vi "Configure Power.vi"(0 "VISA resource name":refnum<visa-resource-name>, 1 "Channel (1)":i32=1, 2 "Port (1)":i32=1, 3 "Port Coupling (T: On)":bool=TRUE, 5 "Power Level (0.0)":dbl format="%^.2g", 7 "Auto Power Range (F: Off)":bool, 9 "Power Range (0.0)":dbl format="%^.2g", 11 "error in (no error)":errorcluster, 12 "Power Slope (F: Off)":bool, 13 "Power Slope Coefficient (0.0)":dbl format="%^.2g") -> (4 "VISA resource name out":refnum<visa-resource-name>, 15 "error out":errorcluster)   [LabVIEW 2018, in "Agilent ENA Series.lvlib"]
doc: "Configures power settings.\n\n<b>Note:</b>\nThis VI is not supported by the E5063A model."
uses:
  Agilent ENA Series.lvlib
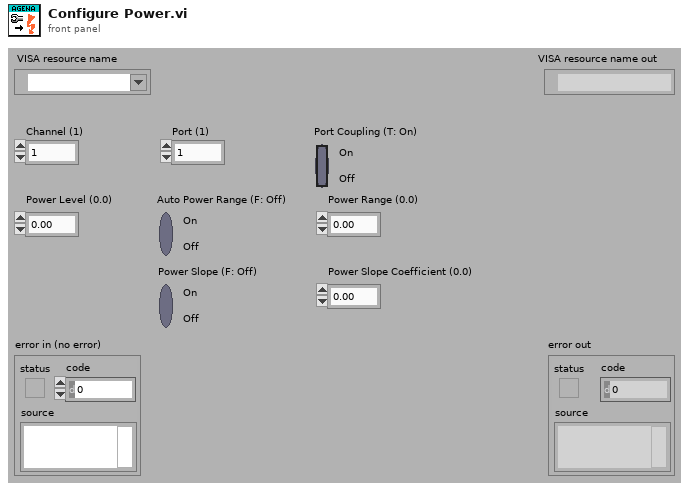
[diagram p1: front panel]
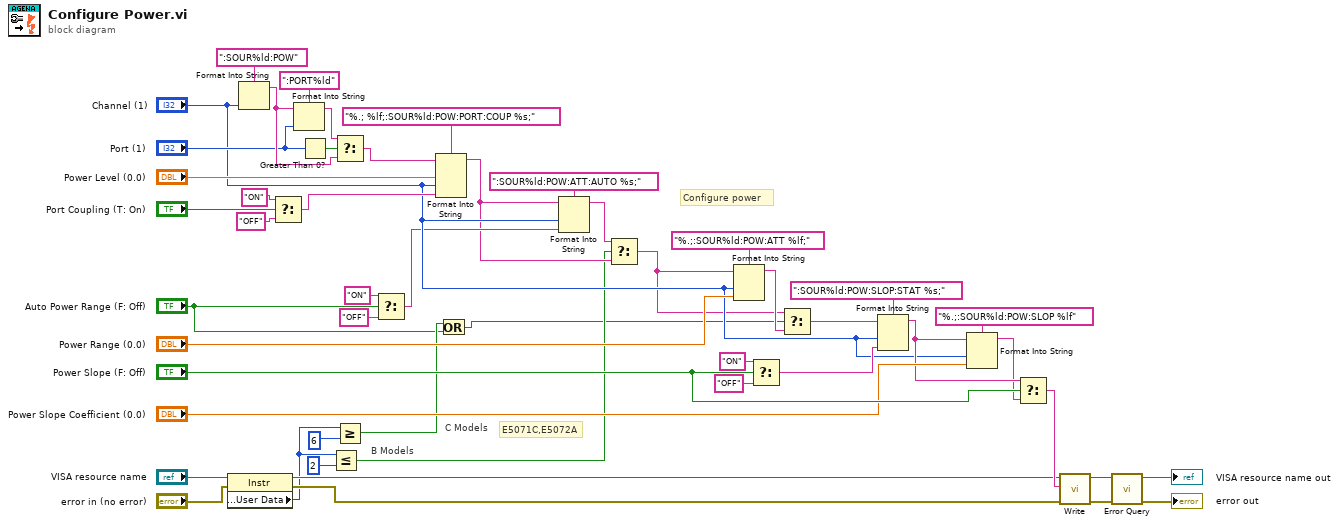
[diagram p0: block diagram]
diagram:
  # "E5071C,E5072A"
  # "Configure power"
  # "C Models"
  # "B Models"
  n1 = property class="Instr"(reference="VISA resource name", error in="error in (no error)") -> (reference out=w15:refnum<visa-resource-name>, error out=w14:errorcluster, "General Settings:User Data"=w2:u32)
  n2 = Format Into String(format string=":SOUR%ld:POW", "Channel (1)") -> (resulting string=w46:string)  [unwired: 2 in, 1 out]
  n3 = Select(t="ON", s="Port Coupling (T: On)", f="OFF") -> (s? t:f=w38:string)
  n4 = Format Into String(format string=":PORT%ld", initial string=w46, "Port (1)") -> (resulting string=w45:string)  [unwired: 1 in, 1 out]
  n5 = Greater Than 0?(x="Port (1)") -> (x > 0?=w47:bool)
  n6 = Less Or Equal?(x=w2, y=u32 2) -> (x <= y?=w7:bool)
  n7 = Select(t=w45, s=w47, f=w46) -> (s? t:f=w43:string)
  n8 = Greater Or Equal?(x=w2, y=u32 6) -> (x >= y?=w5:bool)
  n9 = Select(t="ON", s="Auto Power Range (F: Off)", f="OFF") -> (s? t:f=w12:string)
  n10 = Format Into String(format string="%.; %lf;:SOUR%ld:POW:PORT:COUP %s;", initial string=w43, "Power Level (0.0)", "Channel (1)", w38) -> (resulting string=w8:string)  [unwired: 1 in, 1 out]
  n11 = Or(x=w5, y="Auto Power Range (F: Off)") -> (x .or. y?=w3:bool)
  n12 = Format Into String(format string=":SOUR%ld:POW:ATT:AUTO %s;", initial string=w8, "Channel (1)", w12) -> (resulting string=w9:string)  [unwired: 1 in, 1 out]
  n13 = Select(t=w9, s=w7, f=w8) -> (s? t:f=w10:string)
  n14 = Format Into String(format string="%.;:SOUR%ld:POW:ATT %lf;", initial string=w10, "Channel (1)", "Power Range (0.0)") -> (resulting string=w33:string)  [unwired: 1 in, 1 out]
  n15 = Select(t="ON", s="Power Slope (F: Off)", f="OFF") -> (s? t:f=w28:string)
  n16 = Select(t=w10, s=w3, f=w33) -> (s? t:f=w31:string)
  n17 = Format Into String(format string=":SOUR%ld:POW:SLOP:STAT %s;", initial string=w31, "Channel (1)", w28) -> (resulting string=w24:string)  [unwired: 1 in, 1 out]
  n18 = Format Into String(format string="%.;:SOUR%ld:POW:SLOP %lf", initial string=w24, "Channel (1)", "Power Slope Coefficient (0.0)") -> (resulting string=w23:string)  [unwired: 1 in, 1 out]
  n19 = Select(t=w24, s="Power Slope (F: Off)", f=w23) -> (s? t:f=w22:string)
  n20 = call "Write.vi"("error in (no error)"=w14, "String ()"=w22, "VISA resource name"=w15) -> ("error out"=w20:errorcluster, "VISA resource name out"=w21:refnum<visa-resource-name>)  [unwired: 6 in, 1 out]
  n21 = call "Error Query.vi"("error in (no error)"=w20, "VISA resource name"=w21) -> ("error out"=→"error out":errorcluster, "VISA resource name out"=→"VISA resource name out":refnum<visa-resource-name>)  [unwired: 6 in, 2 out]
